vi "keyboard.vi"() -> ()   [LabVIEW 2014]
panel:
  out "element":dbl
  in  "stop":bool
  in  "Cluster":T1
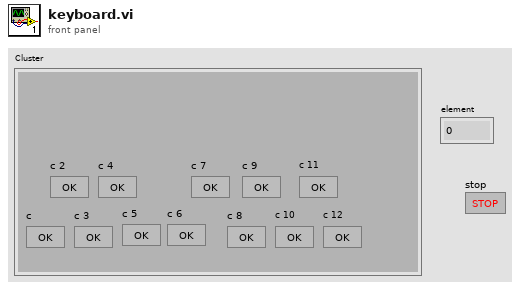
[diagram p1: front panel]
types:
  T1 = cluster{"c":bool, "c 2":bool, "c 3":bool, "c 4":bool, "c 5":bool, "c 6":bool, "c 7":bool, "c 8":bool, "c 9":bool, "c 10":bool, "c 11":bool, "c 12":bool}
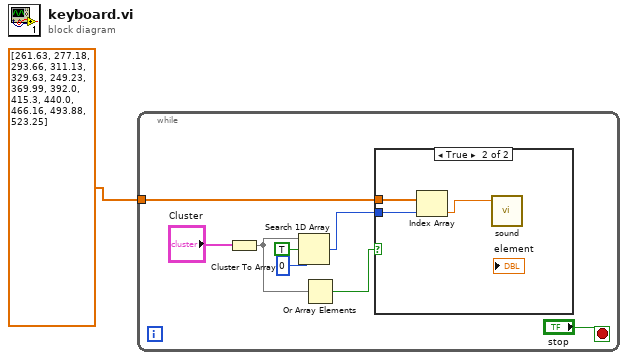
[diagram p0: block diagram]
diagram:
  n1 = while {
    tunnel: dbl[] [261.63, 277.18, 293.66, 311.13, 329.63, 249.23, 369.99, 392.0, 415.3, 440.0, 466.16, 493.88, 523.25] -> [w3]
    stop <- "stop" stop-if-true
    n2 = Cluster To Array(cluster="Cluster") -> (array=w5:bool[])
    n3 = Search 1D Array(1D array=w5, element=TRUE, start index (0)=0) -> (index of element=w2:i32)
    n4 = Or Array Elements(Boolean array=w5) -> (logical OR=w4:bool)
    n5 = case shown="True" w4 {
      tunnel: w3 -> [_ w12]
      tunnel: w2 -> [_ w11]
      frame False {
      }
      frame True {
        n6 = Index Array(array=w12, index=w11) -> (element=w10:dbl)
        n7 = call "sound.vi"("frequency"=w10) -> ()  [unwired: 3 in]
      }
    }
  }
